vi "on_mouse_down.vi"(6 "Mods":cluster{"Double Click":bool, "Menu Key":bool}, 8 "error in (no error)":errorcluster, 9 "Button":u16, 10 "Coords":T1, 11 "window in":refnum<class "rywindow.lvclass">) -> (0 "error out":errorcluster, 3 "window out":refnum<class "rywindow.lvclass">)   [LabVIEW 2017, in "rywindow.lvclass"]
uses:
  rywindow.lvclass
  <vilib>/Utility/miscctls.llb/LVPoint32TypeDef.ctl
  rywindow.lvclass/rywindow.ctl
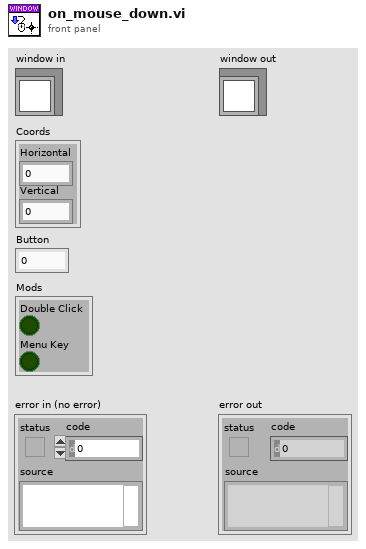
[diagram p1: front panel]
types:
  T1 = typedef "LVPoint32TypeDef.ctl" = cluster{"Horizontal":i32, "Vertical":i32}
  T2 = typedef "LVRowAndColumnTypeDef.ctl" = cluster{"Row":i32, "Column":i32}
  T3 = typedef "rywindow.lvclass/data.ctl" = cluster{"threads":T4[], "MinSize":cluster{"Width":u32, "Height":u32}, "font":T5, "active":i32}
  T4 = typedef "rywindow.lvclass/thread.ctl" = cluster{"name":string, "vi":refnum<vi>}
  T5 = typedef "LVFontTypeDef.ctl" = cluster{"Font Name":string, "Size":u16, "Bold":bool, "Italic":bool, "Underline":bool, "Strikeout":bool, "Color":u32}
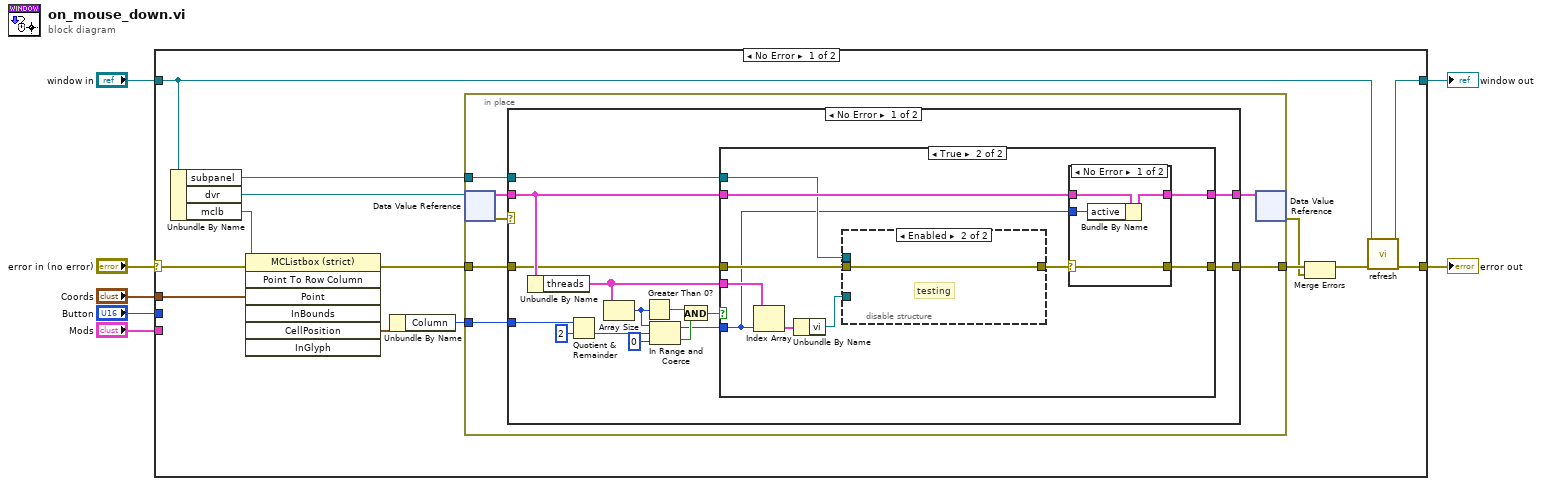
[diagram p0: block diagram]
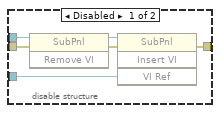
[diagram p4: hidden frame]
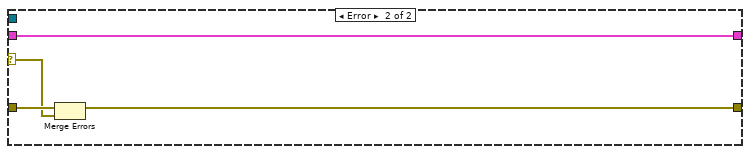
[diagram p5: hidden frame]
diagram:
  n1 = case shown="No Error" "error in (no error)" {
    selector: "error in (no error)" -> [w20 w74]
    tunnel: [w18 w74] -> w6
    tunnel: [w16 w73] -> w4
    tunnel: "window in" -> [w17 w73]
    tunnel: "Coords" -> [w11 _]
    tunnel: "Button" -> [_ _]
    tunnel: "Mods" -> [_ _]
    frame No Error {
      n2 = Unbundle By Name(w17) -> ("subpanel"=w8:refnum<vi>, "dvr"=w21:refnum<data-value>, "mclb"=w12:refnum<vi>)
      n3 = invoke class="MCListbox (strict)" method="Point To Row Column"(reference=w12, error in=w20, "Point"=w11) -> (error out=w13:errorcluster, "CellPosition"=w10:T2)  [unwired: 4 in, 5 out]
      n4 = Unbundle By Name(w10) -> ("Column"=w9:i32)
      n5 = in-place {
        in-place-border: w13 -> [w28]
        in-place-border: [w26] -> w15
        in-place-border: w9 -> [w23]
        in-place-border: w8 -> [w22]
        n6 = in-place-dvr #1(w21) -> (w25:T3, w27:errorcluster)
        n7 = case shown="No Error" w27 {
          selector: w27 -> [_ w70]
          tunnel: w28 -> [w34 w71]
          tunnel: [w33 w69] -> w26
          tunnel: w25 -> [w42 w72]
          tunnel: [w43 w72] -> w24
          tunnel: w23 -> [w31 _]
          tunnel: w22 -> [w32 _]
          frame No Error {
            n8 = Unbundle By Name(w42) -> ("threads"=w37:T4[])
            n9 = Quotient & Remainder(x=w31, y=2) -> (floor(x/y)=w30:i32)  [unwired: 1 out]
            n10 = Array Size(array=w37) -> (size(s)=w40:i32)
            n11 = Greater Than 0?(x=w40) -> (x > 0?=w38:bool)
            n12 = In Range and Coerce(upper limit=w40, x=w30, lower limit=0) -> (coerced(x)=w36:i32, In Range?=w39:bool)
            n13 = And(x=w38, y=w39) -> (x .and. y?=w35:bool)
            n14 = case shown="True" w35 {
              tunnel: [w44 w55] -> w43
              tunnel: w42 -> [w44 w54]
              tunnel: w37 -> [_ w53]
              tunnel: w36 -> [_ w46]
              tunnel: w34 -> [w45 w51]
              tunnel: [w45 w48] -> w33
              tunnel: w32 -> [_ w50]
              frame False {
              }
              frame True {
                n15 = Index Array(array=w53, index=w46) -> (element=w52:T4)
                n16 = Unbundle By Name(w52) -> ("vi"=w49:refnum<vi>)
                n17 = disable-structure shown="Enabled" {
                  disable-tunnel: w51 -> [w67 w68]
                  disable-tunnel: w50 -> [w66 _]
                  disable-tunnel: w49 -> [w63 _]
                  disable-tunnel: [w62 w68] -> w47
                  frame Disabled {
                    n18 = invoke class="SubPnl" method="Remove VI"(reference=w66, error in=w67) -> (reference out=w64:refnum<vi>, error out=w65:errorcluster)  [unwired: 1 in, 1 out]
                    n19 = invoke class="SubPnl" method="Insert VI"(reference=w64, error in=w65, "VI Ref"=w63) -> (error out=w62:errorcluster)  [unwired: 1 in, 3 out]
                  }
                  frame Enabled {
                    # "testing"
                  }
                }
                n20 = case shown="No Error" w47 {
                  selector: w47 -> [w56 w61]
                  tunnel: [w59 w60] -> w55
                  tunnel: w54 -> [w58 w60]
                  tunnel: w46 -> [w57 _]
                  tunnel: [w56 w61] -> w48
                  frame No Error {
                    n21 = Bundle By Name(cluster=w58, "active"=w57) -> (w59:T3)
                  }
                  frame Error {
                  }
                }
              }
            }
          }
          frame Error {
            n22 = Merge Errors(w71, w70) -> (w69:errorcluster)
          }
        }
        n23 = in-place-dvr #1(w24) -> (w14:errorcluster)  [unwired: 1 out]
      }
      n24 = Merge Errors(w15, w14) -> (w19:errorcluster)
      n25 = call "refresh.vi"("error in (no error)"=w19, "window in"=w17) -> ("error out"=w18:errorcluster, "window out"=w16:refnum<class "rywindow.lvclass">)  [unwired: 8 in]
    }
    frame Error {
    }
  }
  "error out" <- w6
  "window out" <- w4
